vi "Fieldscan - save data to file (legacy).vi"(0 "Action":T1, 5 "Magnetic field (T)":dbl, 7 "Lock-in Amplifier (uV)":dbl, 9 "ZVL data array [N segments at constant field]":string[](array[string]), 11 "error in (no error)":errorcluster, 12 "Temperature (K)":dbl) -> (15 "error out":errorcluster)   [LabVIEW 2018]
doc: "Nicolas Weiss - EPFL - IPHYS 2019\n----"
uses:
  Controls/Save data file action.ctl
  Controls/Log destination selector.ctl
  _Global variables 1.vi
panel:
  out "File path":path
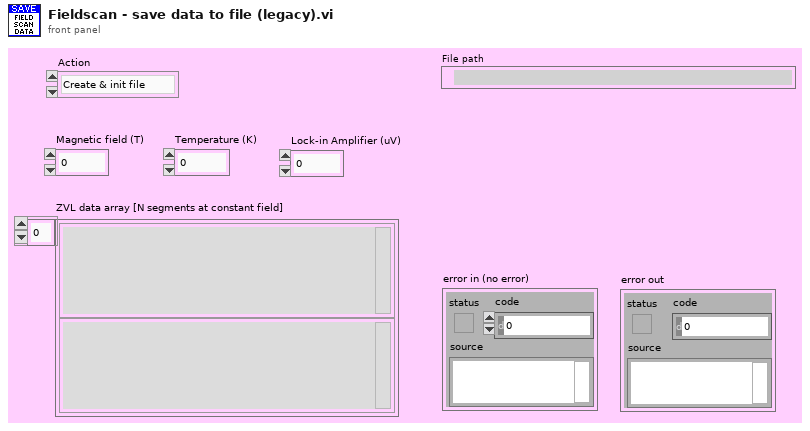
[diagram p1: front panel]
types:
  T1 = typedef "Save data file action.ctl" = enum16{"Create & init file", "Append data", "Close file"}
  T2 = typedef "Log destination selector.ctl" = enum16{"UI", "File", "UI+file"}
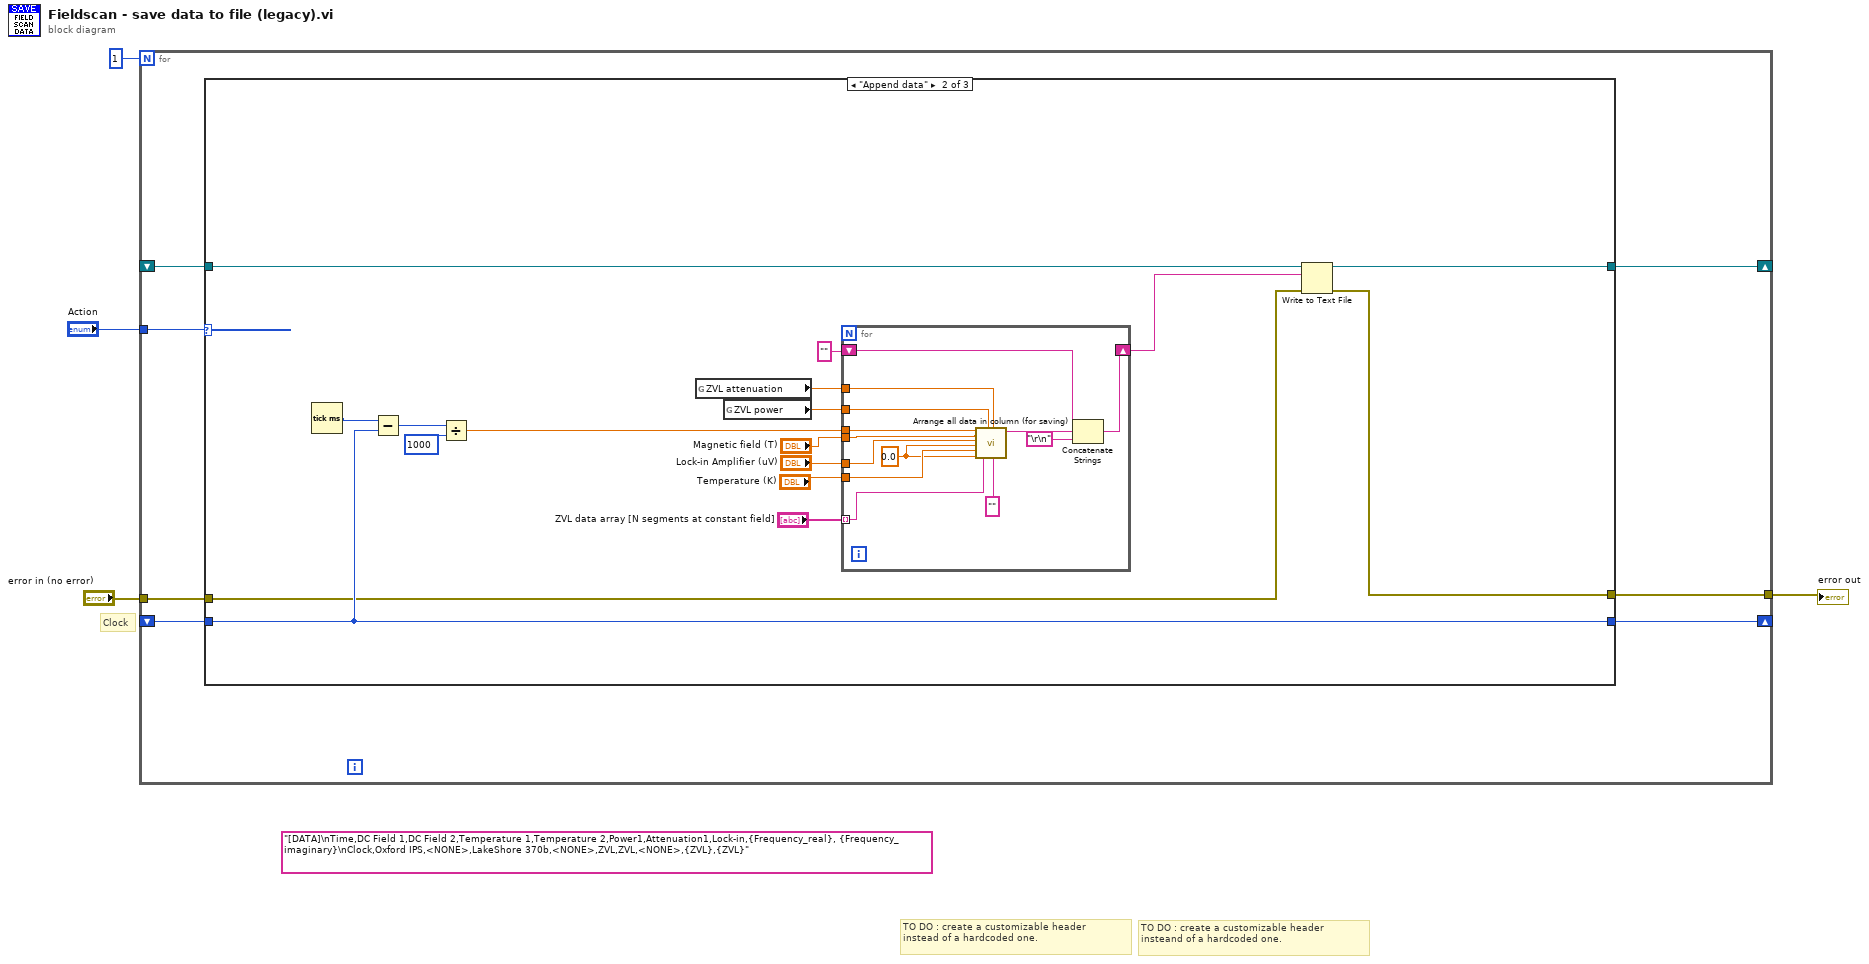
[diagram p0: block diagram]
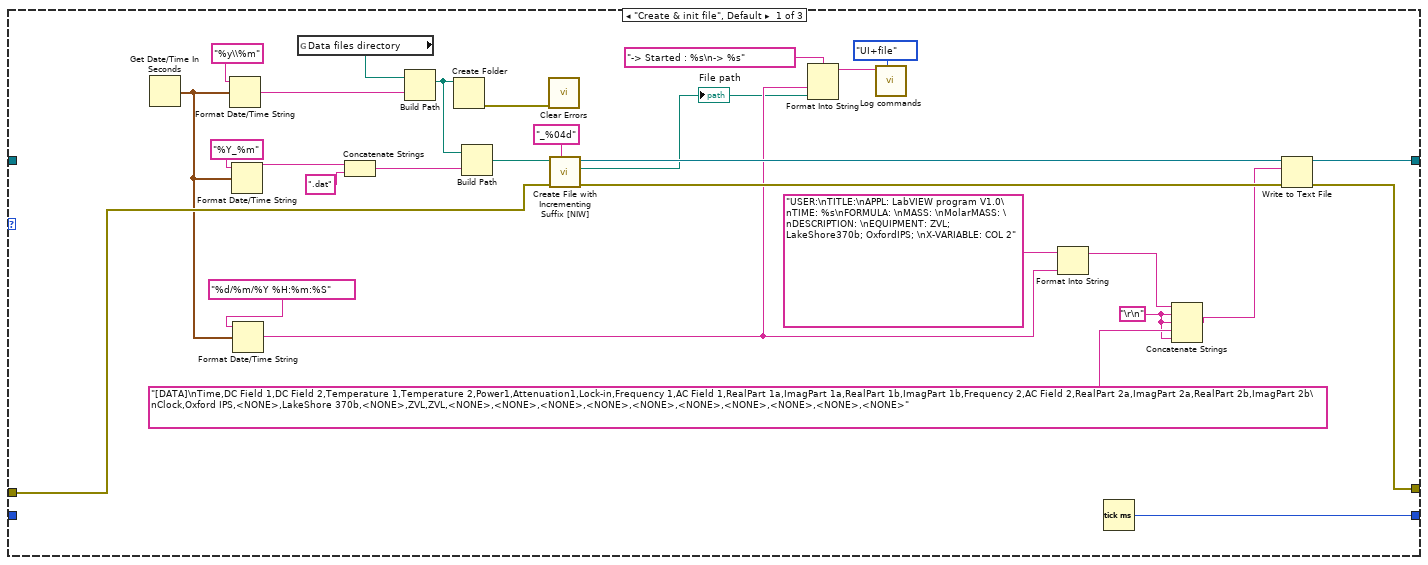
[diagram p2: hidden frame]
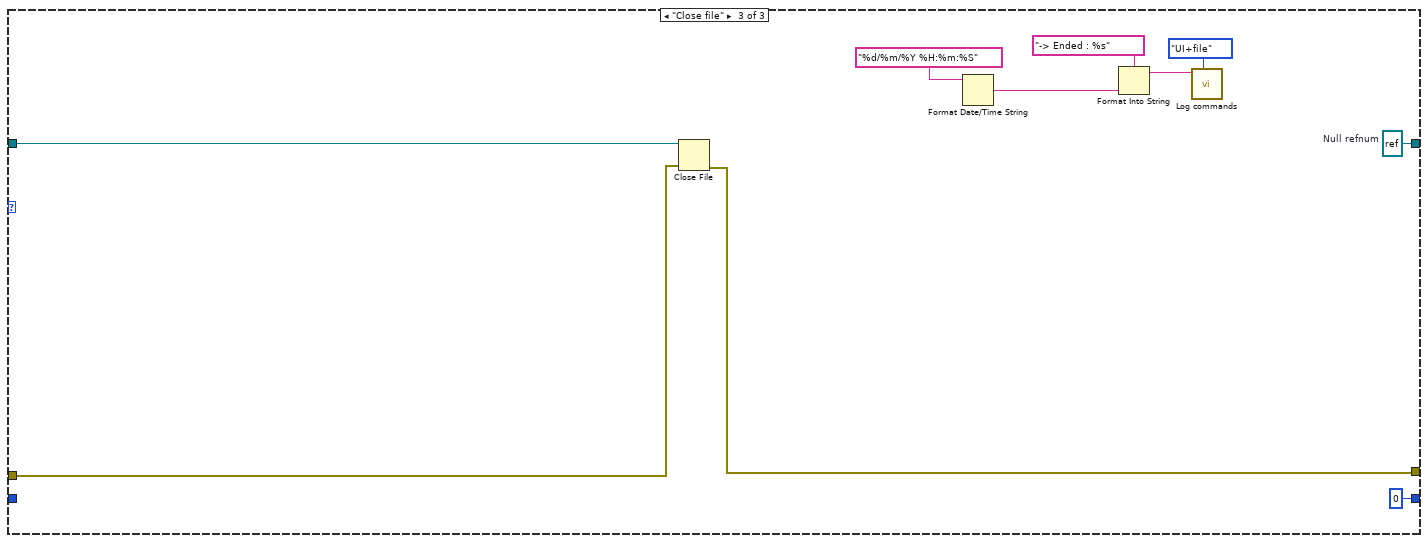
[diagram p3: hidden frame]
diagram:
  (unwired) "[DATA]\nTime,DC Field 1,DC Field 2,Temperature 1,Temperature 2,Power1,Attenuation1,Lock-in,{Frequency_real}, {Frequency_imaginary}\nClock,Oxford IPS,<NONE>,LakeShore 370b,<NONE>,ZVL,ZVL,<NONE>,{ZVL},{ZVL}" ("time format string (%c)")
  # "Clock"
  # "TO DO : create a customizable header \ninsteand of a hardcoded one."
  # "TO DO : create a customizable header \ninstead of a hardcoded one."
  n1 = for {
    N: 1 -> [_]
    shift-right: [w11] -> _
    shift-left: _ -> [w10]
    tunnel: "Action" -> [w9]
    tunnel: "error in (no error)" -> [w8]
    tunnel: [w7] -> w1
    shift-right: [w5] -> _
    shift-left: _ -> [w6]
    n2 = case shown="\"Append data\"" w9 {
      tunnel: [w27 w56 w73] -> w11
      tunnel: w10 -> [_ w57 w80]
      tunnel: w8 -> [w34 w44 w79]
      tunnel: [w25 w43 w78] -> w7
      tunnel: w6 -> [_ w54 _]
      tunnel: [w17 w54 u32 0 ("millisecond timer value")] -> w5
      frame "Create & init file", Default {
        w18 = "\r\n"
        n3 = Get Date/Time In Seconds() -> (seconds since 1Jan1904=w24:timestamp)
        n4 = Format Date/Time String(time format string (%c)="%y\\%m", seconds (now)=w24) -> (date/time string=w38:string)  [unwired: 1 in]
        n5 = Format Date/Time String(time format string (%c)="%Y_%m", seconds (now)=w24) -> (date/time string=w31:string)  [unwired: 1 in]
        n6 = Format Date/Time String(time format string (%c)="%d/%m/%Y %H:%m:%S", seconds (now)=w24) -> (date/time string=w15:string)  [unwired: 1 in]
        n7 = global read "_Global variables 1.vi" "Data files directory"() -> (w39:path)
        n8 = Concatenate Strings(w31, ".dat" ("string")) -> (w29:string)
        n9 = Build Path(base path=w39, name or relative path=w38) -> (appended path=w37:path)
        n10 = Create Folder(path (use dialog)=w37) -> (error out=w36:errorcluster)  [unwired: 2 in, 2 out]
        n11 = Build Path(base path=w37, name or relative path=w29) -> (appended path=w35:path)
        n12 = call <vilib>:"Clear Errors.vi"("error in (no error)"=w36) -> ()  [unwired: 5 in, 2 out]
        n13 = call "Create File with Incrementing Suffix [NIW].vi"("format string (\" (%03d)\")"="_%04d" ("format string (\" (%03d)\")"), "error in (no error)"=w34, "file path"=w35) -> ("error out"=w26:errorcluster, "actual path"=w14:path, "refnum out"=w28:refnum<file>)  [unwired: 5 in, 1 out]
        "File path" <- w14
        n14 = Format Into String(format string="-> Started : %s\n-> %s" ("string"), w15, w14) -> (resulting string=w13:string)  [unwired: 2 in, 1 out]
        n15 = call "Log commands.vi"("Log destination"=Log_destination_selector."UI+file", "text to log"=w13) -> ()  [unwired: 9 in, 1 out]
        n16 = Format Into String(format string="USER:\nTITLE:\nAPPL: LabVIEW program V1.0\nTIME: %s\nFORMULA: \nMASS: \nMolarMASS: \nDESCRIPTION: \nEQUIPMENT: ZVL; LakeShore370b; OxfordIPS; \nX-VARIABLE: COL 2" ("time format string (%c)"), w15) -> (resulting string=w19:string)  [unwired: 2 in, 1 out]
        n17 = Tick Count (ms)() -> (millisecond timer value=w17:u32)
        n18 = Concatenate Strings(w19, w18, w18, "[DATA]\nTime,DC Field 1,DC Field 2,Temperature 1,Temperature 2,Power1,Attenuation1,Lock-in,Frequency 1,AC Field 1,RealPart 1a,ImagPart 1a,RealPart 1b,ImagPart 1b,Frequency 2,AC Field 2,RealPart 2a,ImagPart 2a,RealPart 2b,ImagPart 2b\nClock,Oxford IPS,<NONE>,LakeShore 370b,<NONE>,ZVL,ZVL,<NONE>,<NONE>,<NONE>,<NONE>,<NONE>,<NONE>,<NONE>,<NONE>,<NONE>,<NONE>" ("time format string (%c)"), w18) -> (w21:string)
        n19 = Write to Text File(file (use dialog)=w28, text=w21, error in=w26) -> (refnum out=w27:refnum<file>, error out=w25:errorcluster)  [unwired: 1 in, 1 out]
      }
      frame "Append data" {
        n20 = Tick Count (ms)() -> (millisecond timer value=w55:u32)
        n21 = Subtract(x=w55, y=w54) -> (x-y=w53:u32)
        n22 = Divide(x=w53, y=u32 1000 ("x")) -> (x/y=w51:dbl)
        n23 = global read "_Global variables 1.vi" "ZVL attenuation"() -> (w46:dbl)
        n24 = global read "_Global variables 1.vi" "ZVL power"() -> (w45:dbl)
        n25 = for {
          tunnel: w51 -> [w68]
          tunnel: "Magnetic field (T)" -> [w60]
          tunnel: "Temperature (K)" -> [w67]
          tunnel: "ZVL data array [N segments at constant field]" -> [w65] mode=indexing
          shift-right: [w64] -> w42
          shift-left: "" ("ZVL data 2 [1 segment]") -> [w63]
          tunnel: w46 -> [w62]
          tunnel: w45 -> [w61]
          tunnel: "Lock-in Amplifier (uV)" -> [w58]
          w59 = 0.0 ("Magnetic field 2 (T)")
          n26 = call "Arrange all data in column (for saving).vi"("Time (s)"=w68, "Magnetic field 1 (T)"=w60, "Lock-in Amplifier (uV)"=w58, "Magnetic field 2 (T)"=w59, "Temperature 1 (K)"=w67, "Temperature 2 (K)"=w59, "ZVL data 1 [1 segment]"=w65, "ZVL power (dBm)"=w61, "ZVL attenuation (dB)"=w62, "ZVL data 2 [1 segment]"="") -> ("Result string (for saving)"=w69:string)  [unwired: 9 in]
          n27 = Concatenate Strings(w63, w69, "\r\n") -> (w64:string)
        }
        n28 = Write to Text File(file (use dialog)=w57, text=w42, error in=w44) -> (refnum out=w56:refnum<file>, error out=w43:errorcluster)  [unwired: 1 in, 1 out]
      }
      frame "Close file" {
        w73 = refnum<file> refnum  # Null refnum
        n29 = Close File(refnum=w80, error in=w79) -> (error out=w78:errorcluster)  [unwired: 1 out]
        n30 = Format Date/Time String(time format string (%c)="%d/%m/%Y %H:%m:%S") -> (date/time string=w74:string)  [unwired: 2 in]
        n31 = Format Into String(format string="-> Ended : %s" ("string"), w74) -> (resulting string=w72:string)  [unwired: 2 in, 1 out]
        n32 = call "Log commands.vi"("Log destination"=Log_destination_selector."UI+file", "text to log"=w72) -> ()  [unwired: 9 in, 1 out]
      }
    }
  }
  "error out" <- w1
